vi "UTL_PopulateConfigCtrls.vi"(8 "error in (no error)":errorcluster, 10 "ComConfig":string[](array[string]), 11 "ComNum":i32) -> (0 "error out":errorcluster, 3 "Array Cluster":T1)   [LabVIEW 2019]
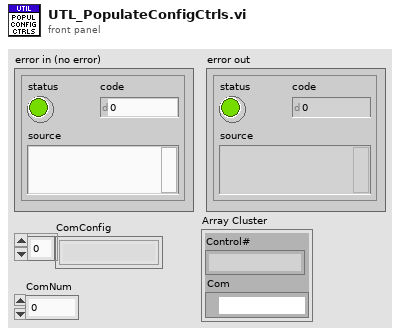
[diagram p1: front panel]
types:
  T1 = cluster{"Control#":string, "Com":refnum<visa-resource-name>}
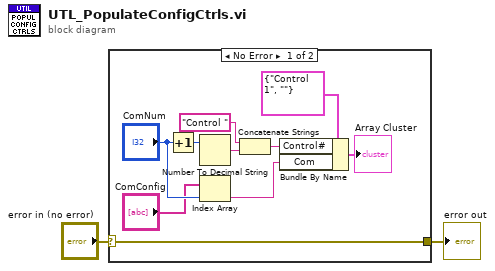
[diagram p0: block diagram]
diagram:
  n1 = case shown="No Error" "error in (no error)" {
    selector: "error in (no error)" -> [w12 w13]
    tunnel: [w12 w13] -> w1
    frame No Error {
      n2 = Increment(x="ComNum") -> (x+1=w7:i32)
      n3 = Number To Decimal String(number=w7) -> (decimal integer string=w11:string)  [unwired: 1 in]
      n4 = Index Array(array="ComConfig", index="ComNum") -> (element=w3:string)
      n5 = Concatenate Strings("Control " ("Control#"), w11) -> (w10:string)
      n6 = Bundle By Name(cluster=T1 {"Control#"="Control 1", "Com"=""} ("CtrlClust"), "Control#"=w10, "Com"=w3) -> (→"Array Cluster":T1)
    }
    frame Error {
    }
  }
  "error out" <- w1
